vi "Read VISA resource name.vi"(8 "Error In":errorcluster, 11 "SerialComm in":refnum<class "SerialComm.lvclass">) -> (0 "Error Out":errorcluster, 2 "VISA Resource":refnum<visa-resource-name>, 3 "SerialComm out":refnum<class "SerialComm.lvclass">)   [LabVIEW 2017, in "SerialComm.lvclass"]
uses:
  SerialComm.lvclass
  SerialComm.lvclass/SerialComm.ctl
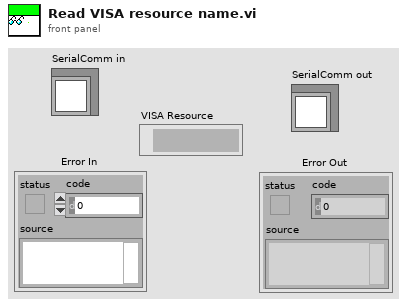
[diagram p1: front panel]
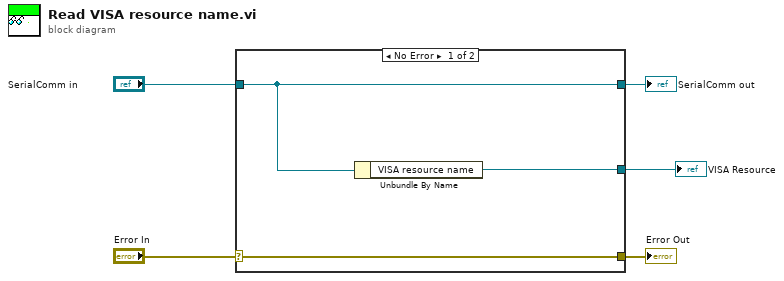
[diagram p0: block diagram]
diagram:
  n1 = case shown="No Error" "Error In" {
    selector: "Error In" -> [w8 w9]
    tunnel: [w8 w9] -> w4
    tunnel: [w7 w10] -> w2
    tunnel: "SerialComm in" -> [w7 w10]
    tunnel: [w6 _] -> w1
    frame No Error {
      n2 = Unbundle By Name(w7) -> ("VISA resource name"=w6:refnum<visa-resource-name>)
    }
    frame Error {
    }
  }
  "Error Out" <- w4
  "SerialComm out" <- w2
  "VISA Resource" <- w1
